vi "jointStatesUnits_roslv.vi"(3 "error in":errorcluster, 4 "Units (deg)":enum16{"Radians", "Degrees"}(ring)=enum."Degrees", 5 "msg in":string) -> (0 "error out":errorcluster, 1 "Joint States":T1(array[cluster]), 2 "msg out":string)   [LabVIEW 2014]
doc: "Parses a message into an array of joint states"
panel:
  out "Header":T2
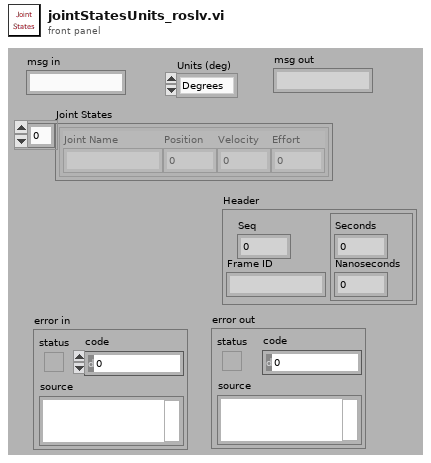
[diagram p1: front panel]
types:
  T1 = cluster{"Joint Name":string, "Position":dbl, "Velocity":dbl, "Effort":dbl}[]
  T2 = cluster{"Seq":u32, "Frame ID":string, cluster{"Seconds":i32, "Nanoseconds":i32}}
  T3 = cluster{"Joint Names":string[], "Position":dbl[], "Velocity":dbl[], "Effort":dbl[]}
  T4 = cluster{"Data to parse":string, "Numeric":dbl, "Numeric":dbl, "Numeric":dbl}
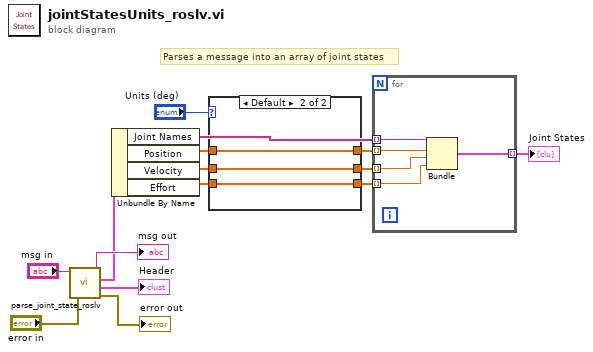
[diagram p0: block diagram]
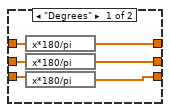
[diagram p2: hidden frame]
diagram:
  # "Parses a message into an array of joint states"
  n1 = call "parse_joint_state_roslv.vi"("error in"="error in", "msg in"="msg in") -> ("error out"=→"error out":errorcluster, "Header"=→"Header":T2, "ROS Joint States"=w9:T3, "msg out"=→"msg out":string)  [unwired: 2 in]
  n2 = Unbundle By Name(w9) -> ("Joint Names"=w5:string[], "Position"=w7:dbl[], "Velocity"=w8:dbl[], "Effort"=w6:dbl[])
  n3 = case shown="Default" "Units (deg)" {
    tunnel: w8 -> [w21 w23]
    tunnel: w7 -> [w20 w24]
    tunnel: w6 -> [w19 w22]
    tunnel: [w18 w24] -> w4
    tunnel: [w17 w23] -> w3
    tunnel: [w16 w22] -> w2
    frame "Degrees" {
      n4 = expression code="x*180/pi"(w20) -> (w18:dbl[])
      n5 = expression code="x*180/pi"(w21) -> (w17:dbl[])
      n6 = expression code="x*180/pi"(w19) -> (w16:dbl[])
    }
    frame Default {
    }
  }
  n7 = for {
    tunnel: w5 -> [w29] mode=indexing
    tunnel: w4 -> [w28] mode=indexing
    tunnel: w3 -> [w27] mode=indexing
    tunnel: w2 -> [w26] mode=indexing
    tunnel: [w25] -> w1 mode=indexing
    n8 = Bundle("Data to parse"=w29, "Numeric"=w28, "Numeric"=w27, "Numeric"=w26) -> (w25:T4)  [unwired: 1 in]
  }
  "Joint States" <- w1
